vi "WSVCAP SHL Host TL SPI Write_Read - Multiple DUTs - Unique Data.vi"(0 "Data Out (Unique)":string[](array[string]), 11 "error in":errorcluster, 13 "DUT Mask (All)":bool[](array[boolean])=[TRUE, TRUE, TRUE, TRUE, TRUE, TRUE, TRUE, TRUE, TRUE, TRUE, TRUE, TRUE, TRUE, TRUE, TRUE, TRUE], 14 "Log (T)":bool=TRUE) -> (4 "SPI Data In":string[](array[string]), 15 "error out":errorcluster)   [LabVIEW 2012]
panel:
  out "SPI Data In [U8]":u8[][](array[numeric]) format="%02x"
  out "Socket Mask":u16=1 format="%02x"
  out "SPI Data Out [U8]":u8[][](array[numeric]) format="%02x"
  # "DUT 01"
  # "DUT 02"
  # "DUT 03"
  # "DUT 04"
  # "DUT 05"
  # "DUT 06"
  # "DUT 07"
  # "DUT 08"
  # "DUT 09"
  # "DUT 10"
  # "DUT 11"
  # "DUT 12"
  # "DUT 13"
  # "DUT 14"
  # "DUT 15"
  # "DUT 16"
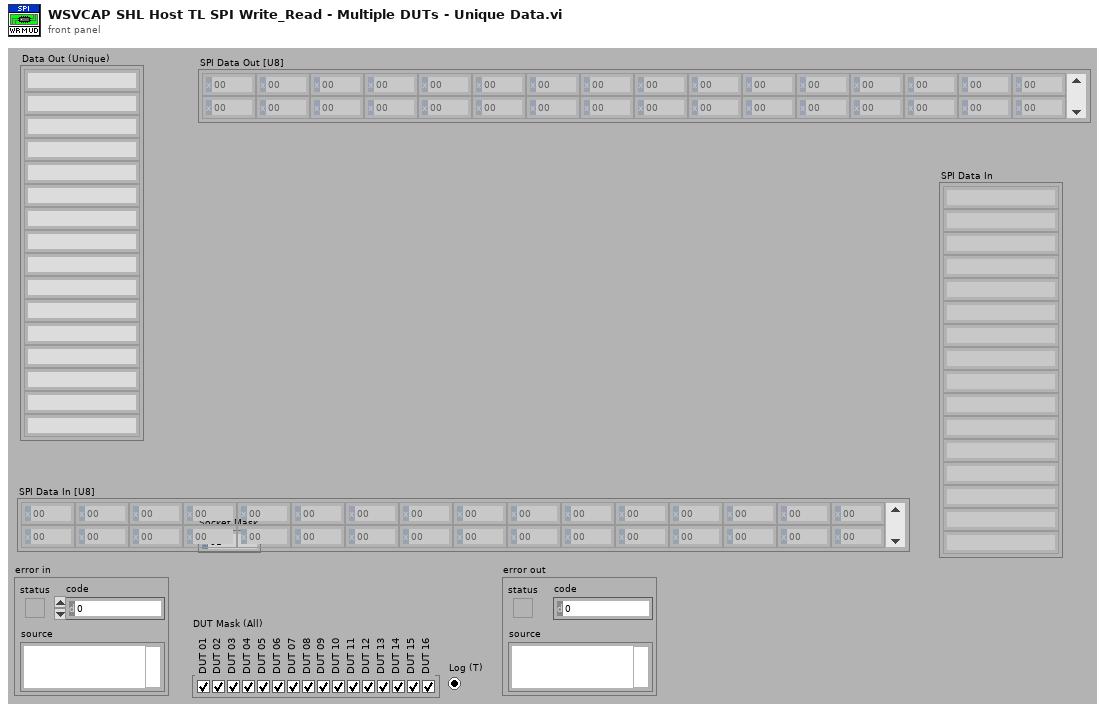
[diagram p1: front panel]
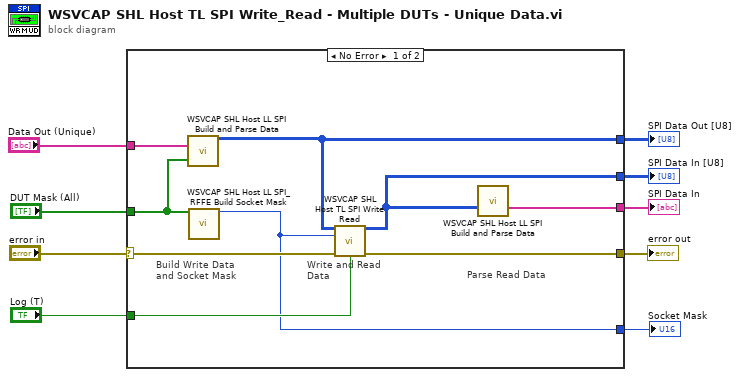
[diagram p0: block diagram]
diagram:
  n1 = case shown="No Error" "error in" {
    selector: "error in" -> [w17 _]
    tunnel: [w18 _] -> w9
    tunnel: "Data Out (Unique)" -> [w15 _]
    tunnel: [w14 _] -> w7
    tunnel: [w12 _] -> w6
    tunnel: "DUT Mask (All)" -> [w16 _]
    tunnel: [w10 _] -> w4
    tunnel: [w11 _] -> w3
    tunnel: "Log (T)" -> [w13 _]
    frame No Error {
      # "Parse Read Data"
      # "Write and Read\nData"
      # "Build Write Data and Socket Mask"
      n2 = call "WSVCAP SHL Host LL SPI Build and Parse Data.vi"("Data Out (Unique)"=w15, "DUT Mask (All)"=w16) -> ("SPI Data Out [U8]"=w14:u8[][])  [unwired: 10 in, 3 out]
      n3 = call "WSVCAP SHL Host LL SPI_RFFE Build Socket Mask.vi"("DUT Mask"=w16) -> ("Socket Mask [U16]"=w12:u16)  [unwired: 13 in, 1 out]
      n4 = call "WSVCAP SHL Host TL SPI Write Read.vi"("SPI Data Out"=w14, "Socket Mask"=w12, "error in"=w17, "Log (T)"=w13) -> ("Read Data Out"=w10:u8[][], "error out"=w18:errorcluster)  [unwired: 10 in]
      n5 = call "WSVCAP SHL Host LL SPI Build and Parse Data.vi"("SPI Data In [U8]"=w10) -> ("SPI Data In"=w11:string[])  [unwired: 11 in, 3 out]
    }
    frame Error {
    }
  }
  "error out" <- w9
  "SPI Data Out [U8]" <- w7
  "Socket Mask" <- w6
  "SPI Data In" <- w3
  "SPI Data In [U8]" <- w4
